vi "5p1_HW_Task2_doanbs.vi"() -> ()   [LabVIEW 2016]
uses:
  <vilib>/express/express arith-compare/Formula/XNode/ExpressFormulaBlockNode.xnode
panel:
  out "Intensity Level":string
  out "MHR (beats/min)":dbl
  in  "Gender (m/f)":string(combo)
  in  "CHR (beats/min)":dbl
  in  "Age (years)":dbl
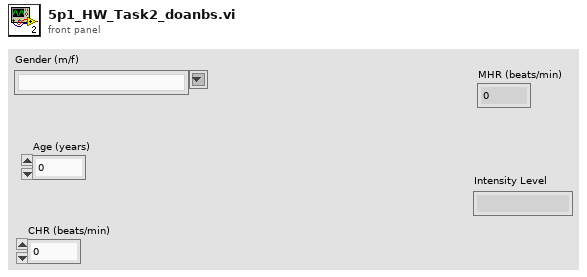
[diagram p1: front panel]
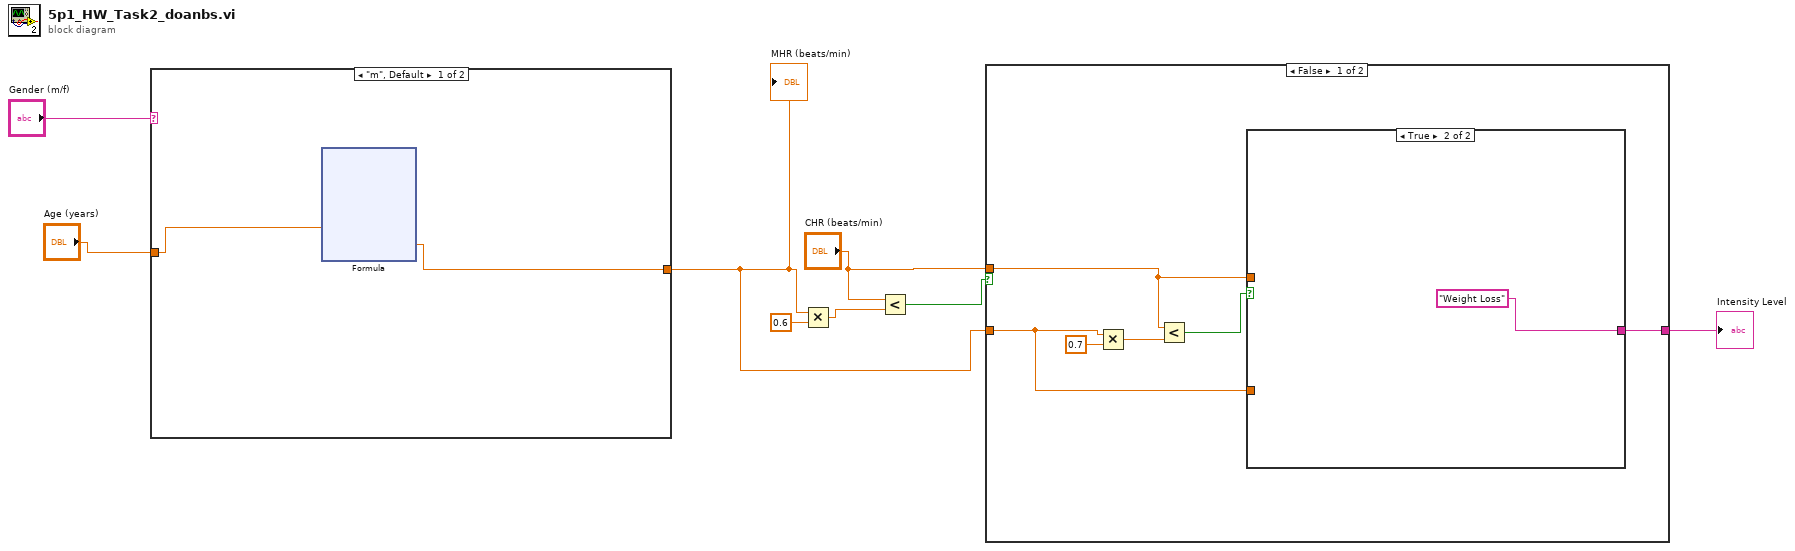
[diagram p0: block diagram]
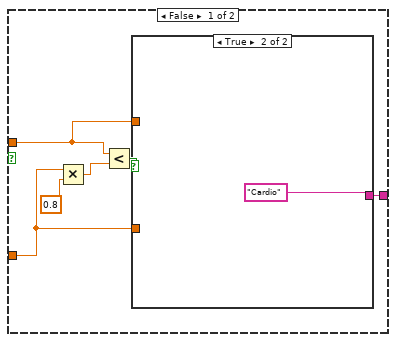
[diagram p2: hidden frame]
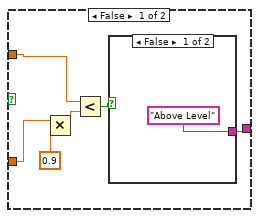
[diagram p3: hidden frame]
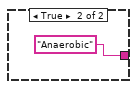
[diagram p4: hidden frame]
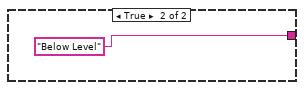
[diagram p5: hidden frame]
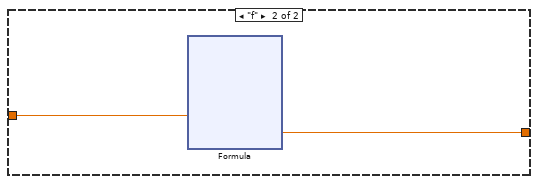
[diagram p6: hidden frame]
diagram:
  n1 = case shown="\"m\", Default" "Gender (m/f)" {
    tunnel: "Age (years)" -> [w10 w20]
    tunnel: [w9 w19] -> w2
    frame "m", Default {
      n2 = xnode "Formula"("a"=w10) -> ("Result"=w9:dbl)  [unwired: 1 in, 1 out]
    }
    frame "f" {
      n3 = xnode "Formula"("a"=w20) -> ("Result"=w19:dbl)  [unwired: 1 in, 1 out]
    }
  }
  "MHR (beats/min)" <- w2
  n4 = Multiply(x=w2, y=0.6) -> (x*y=w4:dbl)
  n5 = Less?(x="CHR (beats/min)", y=w4) -> (x < y?=w6:bool)
  n6 = case shown="False" w6 {
    tunnel: "CHR (beats/min)" -> [w31 _]
    tunnel: w2 -> [w30 _]
    tunnel: [w29 "Below Level"] -> w1
    frame False {
      n7 = Multiply(x=w30, y=0.7) -> (x*y=w33:dbl)
      n8 = Less?(x=w31, y=w33) -> (x < y?=w32:bool)
      n9 = case shown="True" w32 {
        tunnel: w31 -> [w37 _]
        tunnel: w30 -> [w36 _]
        tunnel: [w35 "Weight Loss"] -> w29
        frame False {
          n10 = Multiply(x=w36, y=0.8) -> (x*y=w39:dbl)
          n11 = Less?(x=w37, y=w39) -> (x < y?=w38:bool)
          n12 = case shown="True" w38 {
            tunnel: w37 -> [w43 _]
            tunnel: w36 -> [w42 _]
            tunnel: [w41 "Cardio"] -> w35
            frame False {
              n13 = Multiply(x=w42, y=0.9) -> (x*y=w46:dbl)
              n14 = Less?(x=w43, y=w46) -> (x < y?=w44:bool)
              n15 = case shown="False" w44 {
                tunnel: ["Above Level" "Anaerobic"] -> w41
                frame False {
                }
                frame True {
                }
              }
            }
            frame True {
            }
          }
        }
        frame True {
        }
      }
    }
    frame True {
    }
  }
  "Intensity Level" <- w1
